vi "Depth2ColorImage.vi"(11 "Depth":u16[][](array[numeric])) -> (3 "HSV Image":picture)   [LabVIEW 2015]
uses:
  Control 1.ctl
  <vilib>/picture/picture.llb/Draw True-Color Pixmap.vi
panel:
  out "RHSUS Data Needed":bool
  out "Divisor RHS":dbl
  out "RHS Dist":dbl
  out "LHSUS Data Needed!":bool
  out "CUS Data Needed":bool
  out "Divisor Cent":dbl
  out "Centre Dist":dbl
  out "Divisor LHS":dbl
  out "LHS Dist":dbl
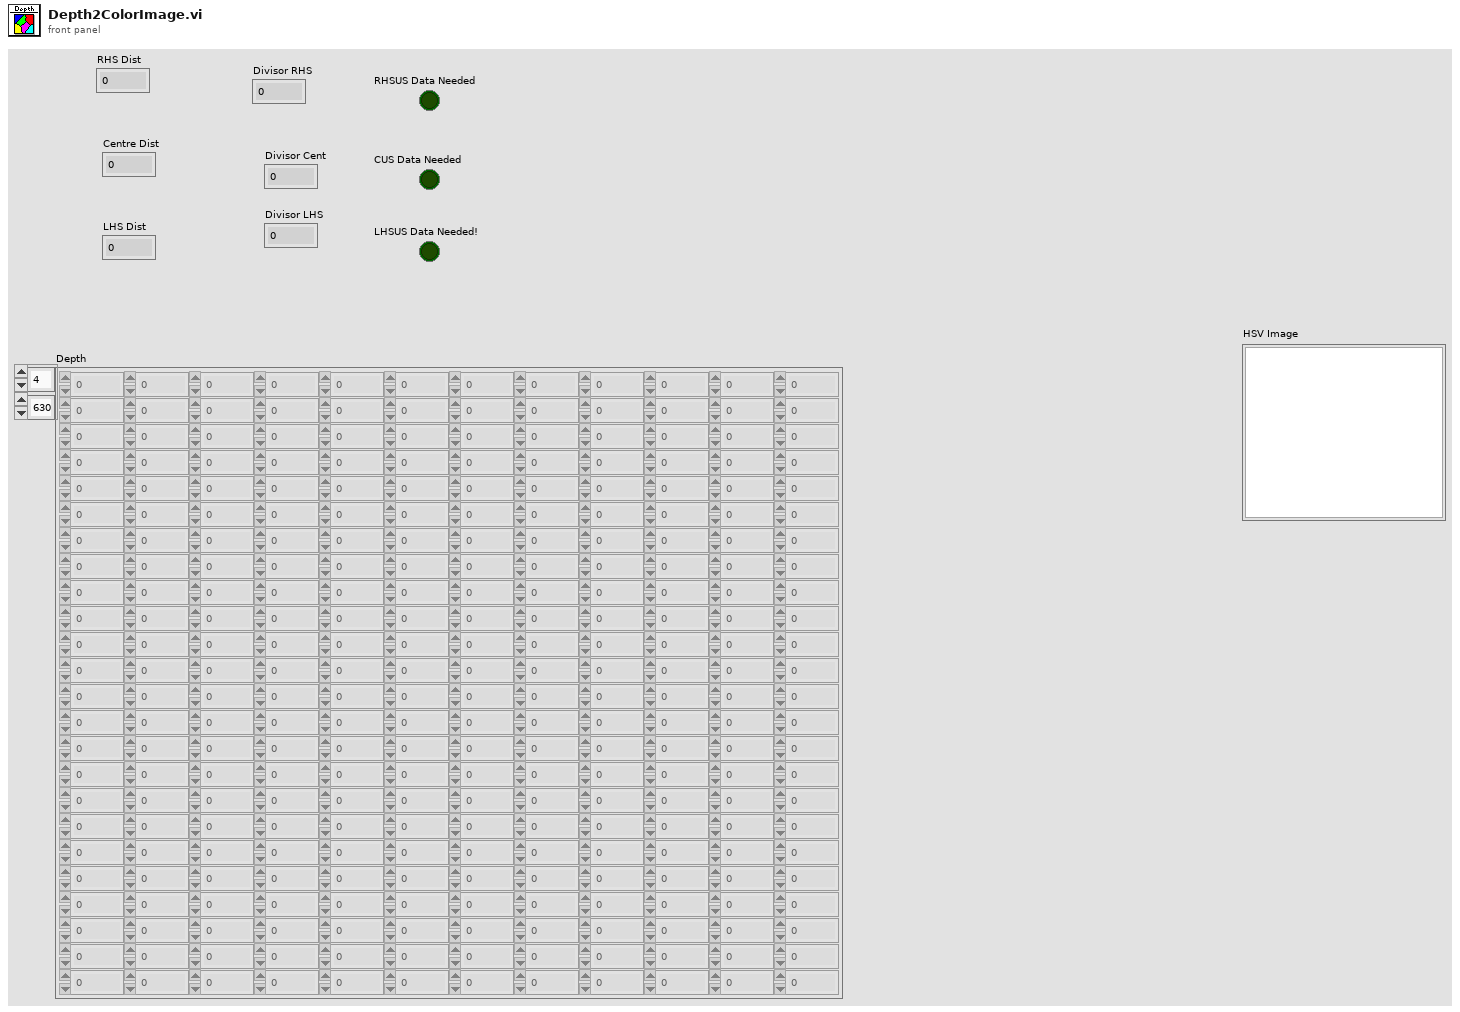
[diagram p1: front panel]
types:
  T1 = typedef "Control 1.ctl" = dbl
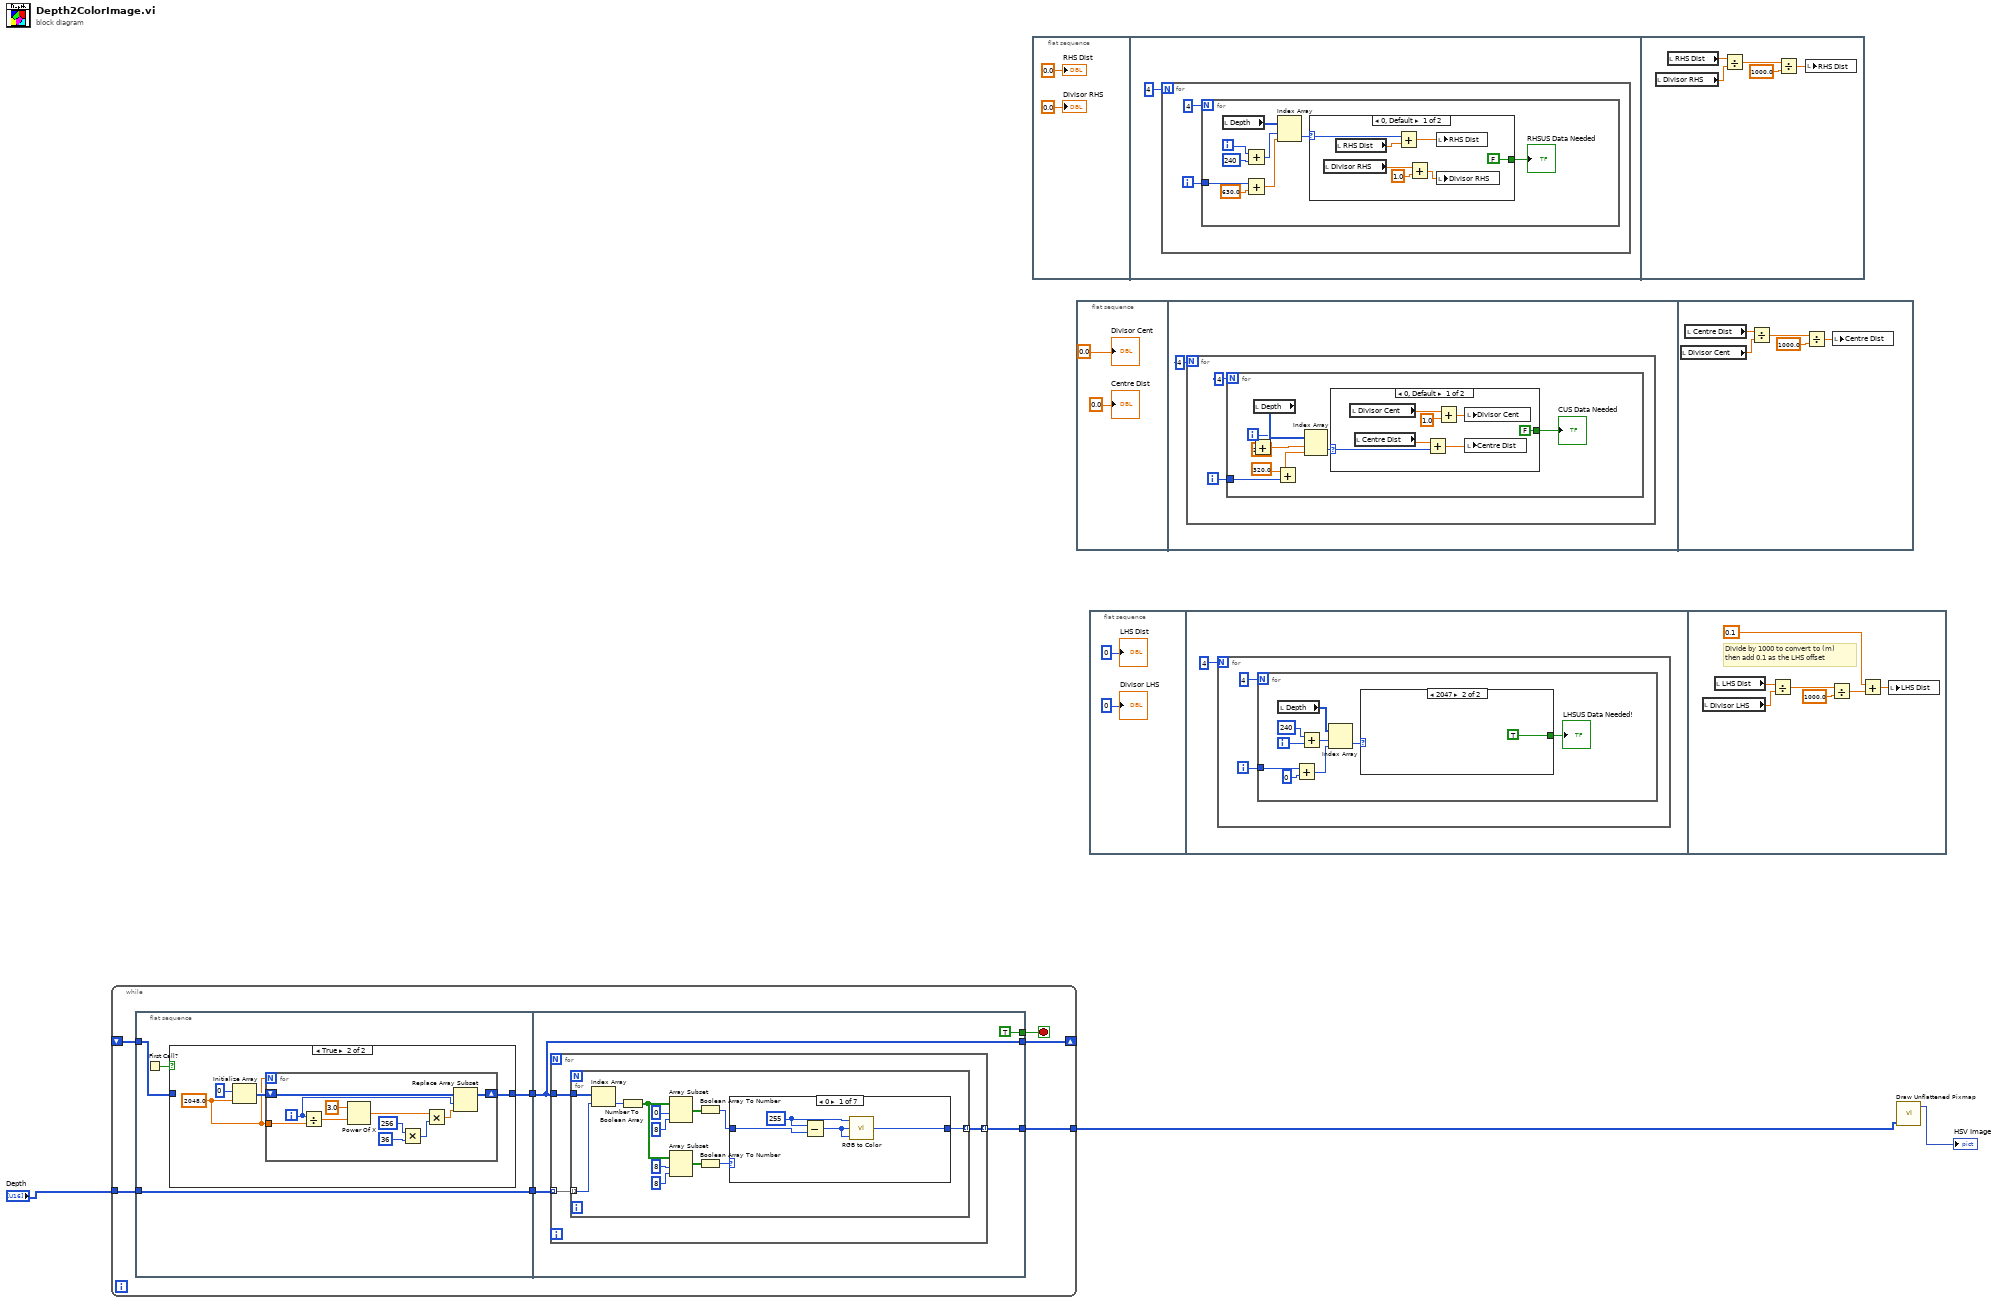
[diagram p0: block diagram]
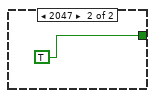
[diagram p2: hidden frame]
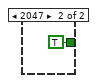
[diagram p3: hidden frame]
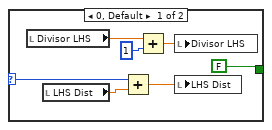
[diagram p4: hidden frame]
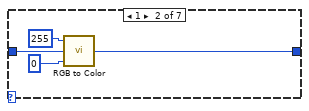
[diagram p6: hidden frame]
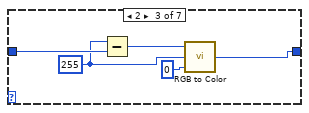
[diagram p7: hidden frame]
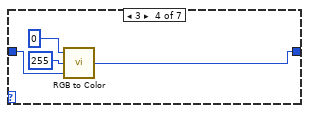
[diagram p8: hidden frame]
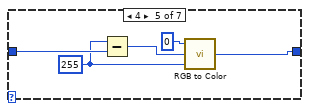
[diagram p9: hidden frame]
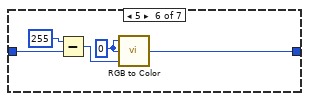
[diagram p10: hidden frame]
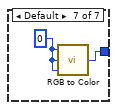
[diagram p11: hidden frame]
diagram:
  n1 = while {
    shift-right: [w9] -> _
    shift-left: _ -> [w8]
    tunnel: "Depth" -> [w6]
    tunnel: [w4] -> w2
    stop <- w5 stop-if-true
    n2 = flat-sequence {
      tunnel: [w13] -> w10
      tunnel: w8 -> [w12]
      tunnel: [w11] -> w7
      tunnel: w6 -> [w11]
      tunnel: w10 -> [w33]
      tunnel: [w33] -> w9
      tunnel: w7 -> [w34]
      tunnel: [TRUE] -> w5
      tunnel: [w31] -> w4
      frame #0 {
        n3 = First Call?() -> (First Call?: T/F=w14:bool)
        n4 = case shown="True" w14 {
          tunnel: [w15 w16] -> w13
          tunnel: w12 -> [w15 _]
          frame False {
          }
          frame True {
            w17 = 2048.0
            n5 = Initialize Array(u16 0 ("element"), w17) -> (w18:u16[])
            n6 = for {
              N: w17 -> [_]
              shift-right: [w21] -> w16
              shift-left: w18 -> [w30]
              tunnel: w17 -> [w28]
              i -> [w29]
              n7 = Divide(x=w29, y=w28) -> (x/y=w27:dbl)
              n8 = Power Of X(1:w27, 2:3.0 ("y")) -> (0:w25:dbl)
              n9 = Multiply(x=256, y=36) -> (x*y=w22:i32)
              n10 = Multiply(x=w25, y=w22) -> (x*y=w20:dbl)
              n11 = Replace Array Subset(array=w30, new element=w20, index=w29) -> (w21:u16[])
            }
          }
        }
      }
      frame #1 {
        n12 = for {
          tunnel: w34 -> [w37] mode=indexing
          tunnel: w33 -> [w36]
          tunnel: [w35] -> w31 mode=indexing
          n13 = for {
            tunnel: w37 -> [w39] mode=indexing
            tunnel: w36 -> [w50]
            tunnel: [w41] -> w35 mode=indexing
            n14 = Index Array(array=w50, index=w39) -> (element=w40:u16)
            n15 = Number To Boolean Array(number=w40) -> (Boolean array=w47:bool[])
            n16 = Array Subset(array=w47, index=0, length=8) -> (w44:bool[])
            n17 = Array Subset(array=w47, index=8, length=8) -> (w43:bool[])
            n18 = Boolean Array To Number(Boolean array=w44) -> (number=w38:u32)
            n19 = Boolean Array To Number(Boolean array=w43) -> (number=w42:u32)
            n20 = case shown="0" w42 {
              tunnel: w38 -> [w53 w56 w63 w64 w70 w76 _]
              tunnel: [w51 w57 w62 w67 w72 w77 w79] -> w41
              frame 0 {
                w54 = 255
                n21 = Subtract(x=w54, y=w53) -> (x-y=w52:u32)
                n22 = call <vilib>:"RGB to Color.vi"("B"=w52, "G"=w52, "R"=w54) -> ("Color"=w51:u32)
              }
              frame 1 {
                n23 = call <vilib>:"RGB to Color.vi"("B"=0, "G"=w56, "R"=255) -> ("Color"=w57:u32)
              }
              frame 2 {
                w60 = 255
                n24 = Subtract(x=w60, y=w63) -> (x-y=w61:u32)
                n25 = call <vilib>:"RGB to Color.vi"("B"=0, "G"=w60, "R"=w61) -> ("Color"=w62:u32)
              }
              frame 3 {
                n26 = call <vilib>:"RGB to Color.vi"("B"=w64, "G"=255, "R"=0) -> ("Color"=w67:u32)
              }
              frame 4 {
                w68 = 255
                n27 = Subtract(x=w68, y=w70) -> (x-y=w69:u32)
                n28 = call <vilib>:"RGB to Color.vi"("B"=w68, "G"=w69, "R"=0) -> ("Color"=w72:u32)
              }
              frame 5 {
                w74 = 0
                n29 = Subtract(x=255, y=w76) -> (x-y=w73:u32)
                n30 = call <vilib>:"RGB to Color.vi"("B"=w73, "G"=w74, "R"=w74) -> ("Color"=w77:u32)
              }
              frame Default {
                w78 = 0
                n31 = call <vilib>:"RGB to Color.vi"("B"=w78, "G"=w78, "R"=w78) -> ("Color"=w79:u32)
              }
            }
          }
        }
      }
    }
  }
  n32 = flat-sequence {
    frame #0 {
      "RHS Dist" <- 0.0 ("RHS Dist")
      "Divisor RHS" <- 0.0 ("Divisor RHS")
    }
    frame #1 {
      n33 = for {
        N: 4 -> [_]
        i -> [w84]
        n34 = for {
          N: 4 -> [_]
          tunnel: w84 -> [w87]
          i -> [w91]
          n35 = local read "Depth"() -> (w93:u16[][])
          n36 = Add(x=w91, y=240) -> (x+y=w92:i32)
          n37 = Add(x=w87, y=630.0) -> (x+y=w89:dbl)
          n38 = Index Array(array=w93, index (row)=w92, index (col)=w89) -> (element=w86:u16)
          n39 = case shown="0, Default" w86 {
            selector: w86 -> [w97 _]
            tunnel: [FALSE TRUE] -> w85
            frame 0, Default {
              n40 = local read "Divisor RHS"() -> (w100:dbl)
              n41 = local read "RHS Dist"() -> (w98:dbl)
              n42 = Add(x=w97, y=w98) -> (x+y=w95:dbl)
              n43 = Add(x=w100, y=1.0) -> (x+y=w96:dbl)
              n44 = local write "RHS Dist"(w95) -> ()
              n45 = local write "Divisor RHS"(w96) -> ()
            }
            frame 2047 {
            }
          }
          "RHSUS Data Needed" <- w85
        }
      }
    }
    frame #2 {
      n46 = local read "Divisor RHS"() -> (w103:dbl)
      n47 = local read "RHS Dist"() -> (w102:dbl)
      n48 = Divide(x=w102, y=w103) -> (x/y=w104:dbl)
      n49 = Divide(x=w104, y=1000.0) -> (x/y=w106:dbl)
      n50 = local write "RHS Dist"(w106) -> ()
    }
  }
  n51 = flat-sequence {
    frame #0 {
      "Centre Dist" <- 0.0 ("Centre Dist")
      "Divisor Cent" <- 0.0 ("Divisor Cent")
    }
    frame #1 {
      n52 = for {
        N: 4 -> [_]
        i -> [w111]
        n53 = for {
          N: 4 -> [_]
          tunnel: w111 -> [w115]
          i -> [w117]
          n54 = Add(x=w117, y=T1 240.0) -> (x+y=w119:T1)
          n55 = local read "Depth"() -> (w120:u16[][])
          n56 = Add(x=320.0, y=w115) -> (x+y=w114:dbl)
          n57 = Index Array(array=w120, index (row)=w119, index (col)=w114) -> (element=w113:u16)
          n58 = case shown="0, Default" w113 {
            selector: w113 -> [w125 _]
            tunnel: [FALSE TRUE] -> w112
            frame 0, Default {
              n59 = local read "Divisor Cent"() -> (w124:dbl)
              n60 = local read "Centre Dist"() -> (w126:dbl)
              n61 = Add(x=w126, y=w125) -> (x+y=w127:dbl)
              n62 = Add(x=w124, y=1.0) -> (x+y=w123:dbl)
              n63 = local write "Divisor Cent"(w123) -> ()
              n64 = local write "Centre Dist"(w127) -> ()
            }
            frame 2047 {
            }
          }
          "CUS Data Needed" <- w112
        }
      }
    }
    frame #2 {
      n65 = local read "Divisor Cent"() -> (w130:dbl)
      n66 = local read "Centre Dist"() -> (w129:dbl)
      n67 = Divide(x=w129, y=w130) -> (x/y=w131:dbl)
      n68 = Divide(x=w131, y=1000.0) -> (x/y=w133:dbl)
      n69 = local write "Centre Dist"(w133) -> ()
    }
  }
  n70 = flat-sequence {
    frame #0 {
      "LHS Dist" <- 0
      "Divisor LHS" <- 0
    }
    frame #1 {
      n71 = for {
        N: 4 -> [_]
        i -> [w137]
        n72 = for {
          N: 4 -> [_]
          tunnel: w137 -> [w142]
          i -> [w146]
          n73 = local read "Depth"() -> (w147:u16[][])
          n74 = Add(x=w142, y=0 ("disabled index (col)")) -> (x+y=w141:i32)
          n75 = Add(x=240 ("index (row)"), y=w146) -> (x+y=w144:i32)
          n76 = Index Array(array=w147, index (row)=w144, index (col)=w141) -> (element=w140:u16)
          n77 = case shown="2047" w140 {
            selector: w140 -> [w154 _]
            tunnel: [FALSE TRUE] -> w139
            frame 0, Default {
              n78 = local read "Divisor LHS"() -> (w151:dbl)
              n79 = local read "LHS Dist"() -> (w153:dbl)
              n80 = Add(x=w154, y=w153) -> (x+y=w152:dbl)
              n81 = Add(x=w151, y=1) -> (x+y=w150:dbl)
              n82 = local write "Divisor LHS"(w150) -> ()
              n83 = local write "LHS Dist"(w152) -> ()
            }
            frame 2047 {
            }
          }
          "LHSUS Data Needed!" <- w139
        }
      }
    }
    frame #2 {
      # "Divide by 1000 to convert to (m) \nthen add 0.1 as the LHS offset"
      n84 = local read "Divisor LHS"() -> (w162:dbl)
      n85 = local read "LHS Dist"() -> (w161:dbl)
      n86 = Divide(x=w161, y=w162) -> (x/y=w160:dbl)
      n87 = Divide(x=w160, y=1000.0) -> (x/y=w157:dbl)
      n88 = Add(x=0.1, y=w157) -> (x+y=w158:dbl)
      n89 = local write "LHS Dist"(w158) -> ()
    }
  }
  n90 = call-poly <vilib>:"Draw Unflattened Pixmap.vi"("data (RGB format)"=w2) -> ("new picture"=→"HSV Image":picture)  [unwired: 8 in]
